vi "Samsung Data String.vi"(10 "# Racks":i32=1, 11 "Samsung Data In":u16[](array[numeric])) -> (2 "Contactor CMD":bool[](array[boolean]), 3 "Samsung String Data Array":T1[](array[typedef]))   [LabVIEW 2014]
uses:
  Controls/ES String Data.ctl
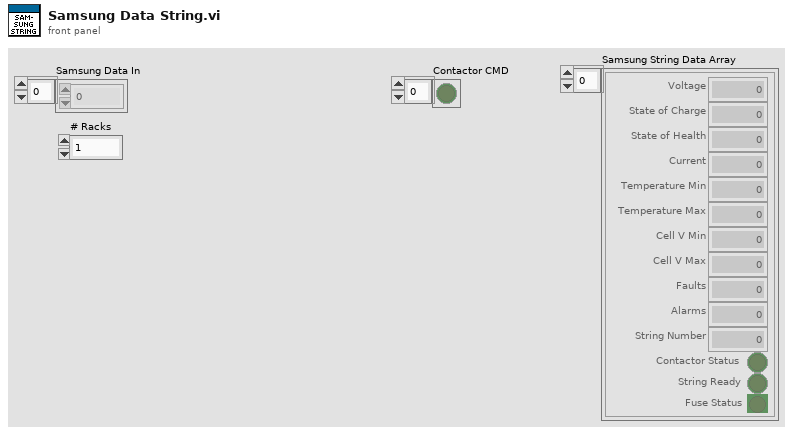
[diagram p1: front panel]
types:
  T1 = typedef "ES String Data.ctl" = cluster{"Voltage":sgl, "State of Charge":sgl, "Current":sgl, "Temperature Min":i16, "Temperature Max":i16, "Faults":u16, "Alarms":u16, "String Number":u16, "Contactor Status":bool, "String Ready":bool, "Fuse Status":bool, "Cell V Max":dbl, "Cell V Min":dbl, "State of Health":sgl}
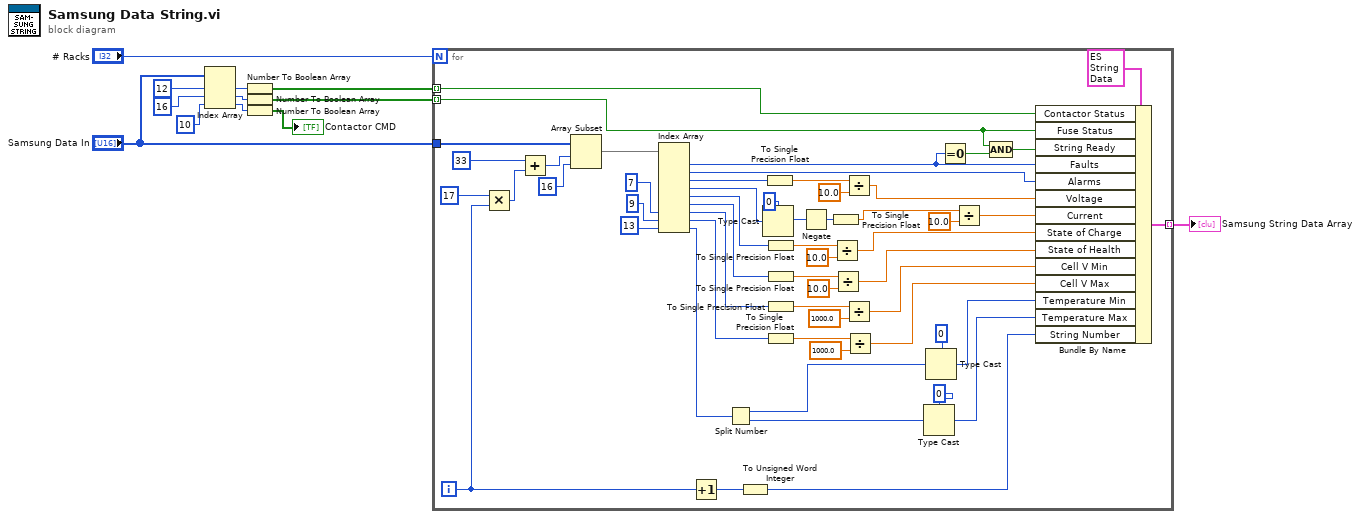
[diagram p0: block diagram]
diagram:
  n1 = Index Array(array="Samsung Data In", index #1=12 ("index"), index #2=16 ("index"), index #3=10 ("index")) -> (element #1=w11:u16, element #2=w5:u16, element #3=w2:u16)
  n2 = Number To Boolean Array(number=w11) -> (Boolean array=w9:bool[])
  n3 = Number To Boolean Array(number=w5) -> (Boolean array=w4:bool[])
  n4 = Number To Boolean Array(number=w2) -> (Boolean array=→"Contactor CMD":bool[])
  n5 = for {
    N: "# Racks" -> [_]
    tunnel: w9 -> [w16] mode=indexing
    tunnel: [w60] -> w7 mode=indexing
    tunnel: "Samsung Data In" -> [w36]
    tunnel: w4 -> [w13] mode=indexing
    i -> [w31]
    n6 = Multiply(x=17, y=w31) -> (x*y=w32:i32)
    n7 = Add(x=33 ("index"), y=w32) -> (x+y=w34:i32)
    n8 = Array Subset(array=w36, index=w34, length=16) -> (w35:u16[])
    n9 = Index Array(array=w35, index #7=7 ("index"), index #8=9 ("index"), index #9=13 ("index")) -> (element #1=w29:u16, element #2=w65:u16, element #3=w49:u16, element #4=w50:u16, element #5=w51:u16, element #6=w19:u16, element #7=w24:u16, element #8=w23:u16, element #9=w22:u16)  [unwired: 6 in]
    n10 = Increment(x=w31) -> (x+1=w66:i32)
    n11 = Split Number(x=w22) -> (hi(x)=w62:u8, lo(x)=w61:u8)
    n12 = To Unsigned Word Integer(number=w66) -> (unsigned 16bit integer=w17:u16)
    n13 = Type Cast(type=i16 0, x=w50) -> (*(type *) &x=w48:i16)
    n14 = To Single Precision Float(number=w49) -> (single precision float=w57:sgl)
    n15 = To Single Precision Float(number=w51) -> (single precision float=w55:sgl)
    n16 = To Single Precision Float(number=w19) -> (single precision float=w20:sgl)
    n17 = To Single Precision Float(number=w24) -> (single precision float=w41:sgl)
    n18 = To Single Precision Float(number=w23) -> (single precision float=w39:sgl)
    n19 = Negate(x=w48) -> (-x=w54:i16)
    n20 = To Single Precision Float(number=w54) -> (single precision float=w52:sgl)
    n21 = Divide(x=w55, y=sgl 10.0) -> (x/y=w44:sgl)
    n22 = Divide(x=w20, y=sgl 10.0) -> (x/y=w18:sgl)
    n23 = Divide(x=w57, y=sgl 10.0) -> (x/y=w45:sgl)
    n24 = Divide(x=w41, y=sgl 1000.0) -> (x/y=w28:sgl)
    n25 = Divide(x=w39, y=sgl 1000.0) -> (x/y=w38:sgl)
    n26 = Type Cast(type=i8 0 ("y"), x=w61) -> (*(type *) &x=w59:i8)
    n27 = Type Cast(type=i8 0 ("y"), x=w62) -> (*(type *) &x=w43:i8)
    n28 = Equal To 0?(x=w29) -> (x = 0?=w15:bool)
    n29 = Divide(x=w52, y=sgl 10.0) -> (x/y=w46:sgl)
    n30 = Compound Arithmetic op=AND(w13, w15) -> (w14:bool)
    n31 = Bundle By Name(cluster=T1 {"Voltage"=0.0, "State of Charge"=0.0, "Current"=0.0, "Temperature Min"=0, "Temperature Max"=0, "Faults"=0, "Alarms"=0, "String Number"=0, "Contactor Status"=FALSE, "String Ready"=FALSE, "Fuse Status"=FALSE, "Cell V Max"=0.0, "Cell V Min"=0.0, "State of Health"=0.0} ("Energy Storage String Data"), "Contactor Status"=w16, "Fuse Status"=w13, "String Ready"=w14, "Faults"=w29, "Alarms"=w65, "Voltage"=w45, "Current"=w46, "State of Charge"=w44, "State of Health"=w18, "Cell V Min"=w28, "Cell V Max"=w38, "Temperature Min"=w43, "Temperature Max"=w59, "String Number"=w17) -> (w60:T1)
  }
  "Samsung String Data Array" <- w7
